vi "02 -  Clever Debugging.vi"() -> ()   [LabVIEW 2021]
uses:
  <vilib>/Analysis/NI_AALBase.lvlib
  0321a4c6-245a-4374-bf8e-c30a36aea294.vi
panel:
  in  "Stop Button":bool
  in  "dequeue delay, ms":u32
  in  "enqueue interval, ms":u32=15
  # "Open Block Diagram to Debug Code\nCtl + E (instructions on diagram)"
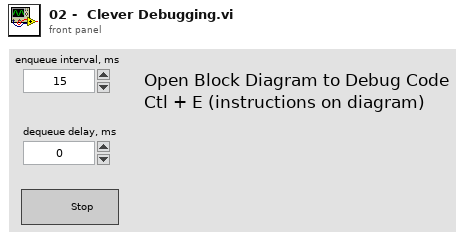
[diagram p1: front panel]
types:
  T1 = enum16{"open", "replace", "create", "open or create", "replace or create", "replace or create with confirmation"}
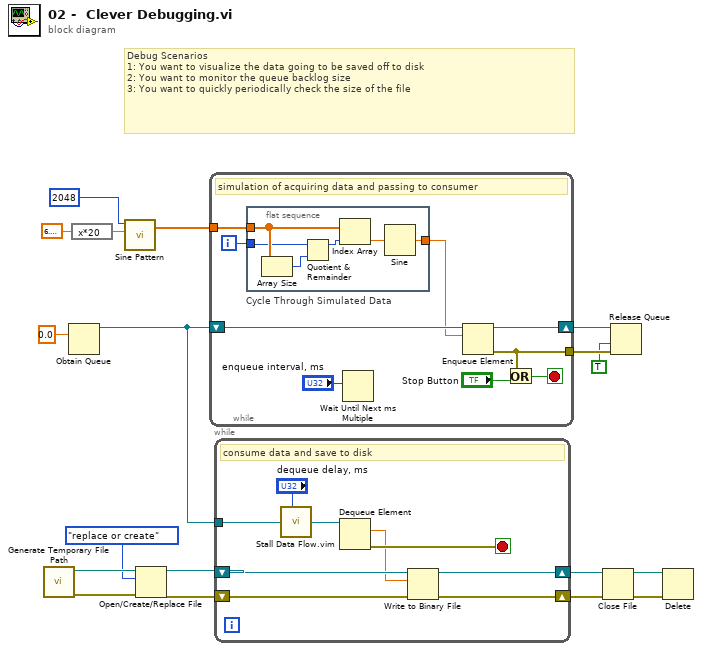
[diagram p0: block diagram]
diagram:
  # "Debug Scenarios\n1: You want to visualize the data going to be saved off to disk\n2: You want to monitor the queue backlog size\n3: You want to quickly periodically check the size of the file"
  n1 = call <vilib>:"Generate Temporary File Path.vi"() -> ("error out"=w11:errorcluster, "Unique Temporary File Path"=w12:path)  [unwired: 10 in]
  n2 = Obtain Queue(element data type=0.0 ("sin(x)")) -> (queue out=w18:refnum<queue>)  [unwired: 4 in, 2 out]
  n3 = expression code="x*20"(6.283185307179586) -> (w14:dbl)
  n4 = call <vilib>:"Sine Pattern.vi"("amplitude"=w14, "samples"=2048) -> ("Sinusoidal Pattern"=w17:dbl[])  [unwired: 2 in, 1 out]
  n5 = Open/Create/Replace File(file path (use dialog)=w12, error in=w11, operation (0:open)=T1."replace or create") -> (refnum out=w10:refnum<file>, error out=w9:errorcluster)  [unwired: 3 in, 1 out]
  n6 = while {
    tunnel: w17 -> [w26]
    tunnel: [w20] -> w2
    shift-right: [w21] -> w3
    shift-left: w18 -> [w27]
    i -> [w19]
    stop <- w22 stop-if-true
    # "simulation of acquiring data and passing to consumer"
    n7 = flat-sequence "Cycle Through Simulated Data" {
      tunnel: w19 -> [w28]
      tunnel: w26 -> [w32]
      tunnel: [w30] -> w25
      frame #0 {
        n8 = Array Size(array=w32) -> (size(s)=w29:i32)
        n9 = Quotient & Remainder(x=w28, y=w29) -> (x-y*floor(x/y)=w33:i32)  [unwired: 1 out]
        n10 = Index Array(array=w32, index=w33) -> (element=w31:dbl)
        n11 = Sine(x=w31) -> (sin(x)=w30:dbl)
      }
    }
    n12 = Wait Until Next ms Multiple(millisecond multiple="enqueue interval, ms") -> ()  [unwired: 1 out]
    n13 = Enqueue Element(queue=w27, element=w25) -> (queue out=w21:refnum<queue>, error out=w20:errorcluster)  [unwired: 2 in, 1 out]
    n14 = Or(x=w20, y="Stop Button") -> (x .or. y?=w22:bool)
  }
  n15 = while {
    tunnel: w18 -> [w42]
    shift-right: [w36] -> w8
    shift-left: w10 -> [w38]
    shift-right: [w35] -> w7
    shift-left: w9 -> [w37]
    stop <- w41 stop-if-true
    # "consume data and save to disk"
    n16 = call "Stall Data Flow.vim"("value in"=w42, "milliseconds to wait"="dequeue delay, ms") -> ("value out"=w40:refnum<queue>)  [unwired: 1 out]
    n17 = Dequeue Element(queue=w40) -> (element=w34:dbl, error out=w41:errorcluster)  [unwired: 2 in, 2 out]
    n18 = Write to Binary File(file (use dialog)=w38, data=w34, error in=w37) -> (refnum out=w36:refnum<file>, error out=w35:errorcluster)  [unwired: 3 in, 1 out]
  }
  n19 = Close File(refnum=w8, error in=w7) -> (path=w5:path, error out=w6:errorcluster)
  n20 = Release Queue(queue=w3, force destroy? (F)=TRUE, error in (no error)=w2) -> ()  [unwired: 3 out]
  n21 = Delete(path (use dialog)=w5, error in=w6) -> ()  [unwired: 3 in, 3 out]
